vi "ReadOrWriteToJSONfile.vi"(7 "Data":T1, 8 "error in (no error)":errorcluster, 10 "Command":enum16{"Read", "Write"}(ring), 11 "JSONtext Input":string) -> (0 "error out":errorcluster, 3 "JSON text":string)   [LabVIEW 2017]
doc: "<B>This VI is used for Read or Write a JSON file.</B>"
uses:
  <vilib>/JDP Science/JSONtext/JSONtext.lvlib
  Ctrl/Property.ctl
  Ctrl/PhysicalChannel.ctl
  Ctrl/Bitfield.ctl
  Ctrl/Register.ctl
  Ctrl/ScaleType.ctl
  Ctrl/Scale.ctl
  Ctrl/EnumValue.ctl
  Ctrl/Enum.ctl
  Ctrl/Caps.ctl
  Ctrl/Data.ctl
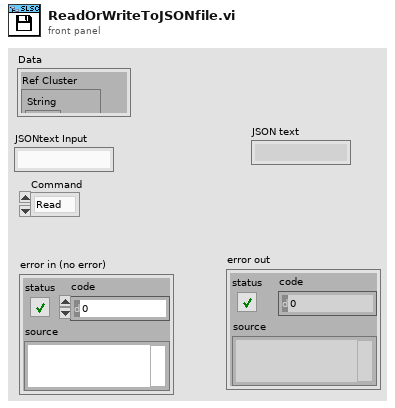
[diagram p1: front panel]
types:
  T1 = typedef "Data.ctl" = cluster{"Ref Cluster":cluster{"String":refnum<vi>, "U8":refnum<vi>, "I8":refnum<vi>, "U32":refnum<vi>, "I32":refnum<vi>, "U64":refnum<vi>, "I64":refnum<vi>, "Ring":refnum<vi>, "DBL":refnum<vi>, "Add":refnum<vi>, "Remove":refnum<vi>, "Property tree":refnum<vi>, "confirm":refnum<vi>}, "JSON Text":string, "Original JSON Text":string, "Caps":T2, "SLSC Output Tree":cluster{"Left Cell String":string, "Child Text":string[], "Child Tag":string, "Item Indent":i32, "Child Only?":bool, "Glyph Index":i32, "offline value":variant}[], "Ref Index and Control Type":cluster{"index":i32, "Datatype":string}, "Selected Type and name":cluster{"Selected Type":enum16{"Property", "Physical Channel", "Other"}, "Selected Property Name":string}, "Update whole Tree?":bool}
  T2 = typedef "Caps.ctl" = cluster{"properties":T3[], "physical channels":T4[], "registers":T5[], "scales":T7[], "enums":T9[], "productName":string}
  T3 = typedef "Property.ctl" = cluster{"name":string, "bitfield":string, "value":variant, "dataType":string, "min":variant, "max":variant, "scale":string, "access":string}
  T4 = typedef "PhysicalChannel.ctl" = cluster{"name":string, "properties":T3[]}
  T5 = typedef "Register.ctl" = cluster{"name":string, "address":i32, "size":i32, "bitfields":T6[], "initialValue":variant, "connectedProperties":string[]}
  T6 = typedef "Bitfield.ctl" = cluster{"name":string, "offset":i32, "size":i32, "signed":bool}
  T7 = typedef "Scale.ctl" = cluster{"name":string, "type":T8, "params":variant}
  T8 = typedef "ScaleType.ctl" = enum16{"NoScale", "Table", "Polynomial", "Linear"}
  T9 = typedef "Enum.ctl" = cluster{"name":string, "values":T10[]}
  T10 = typedef "EnumValue.ctl" = cluster{"name":string, "value":i32}
  T11 = enum16{"open", "replace", "create", "open or create", "replace or create", "replace or create with confirmation"}
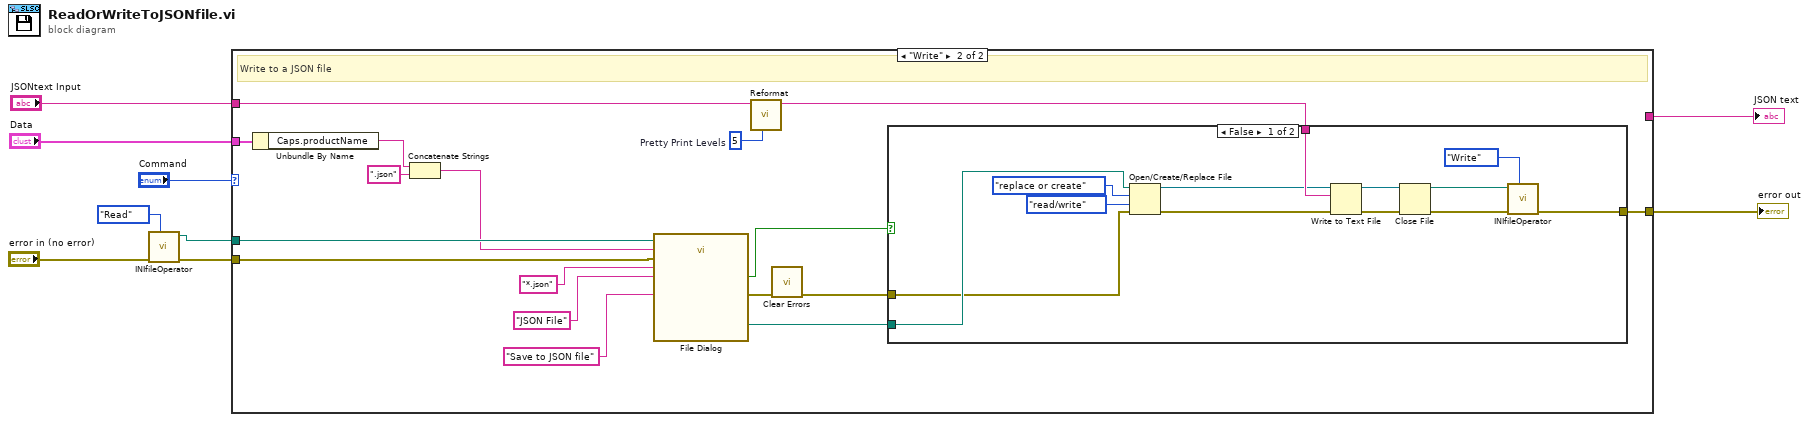
[diagram p0: block diagram]
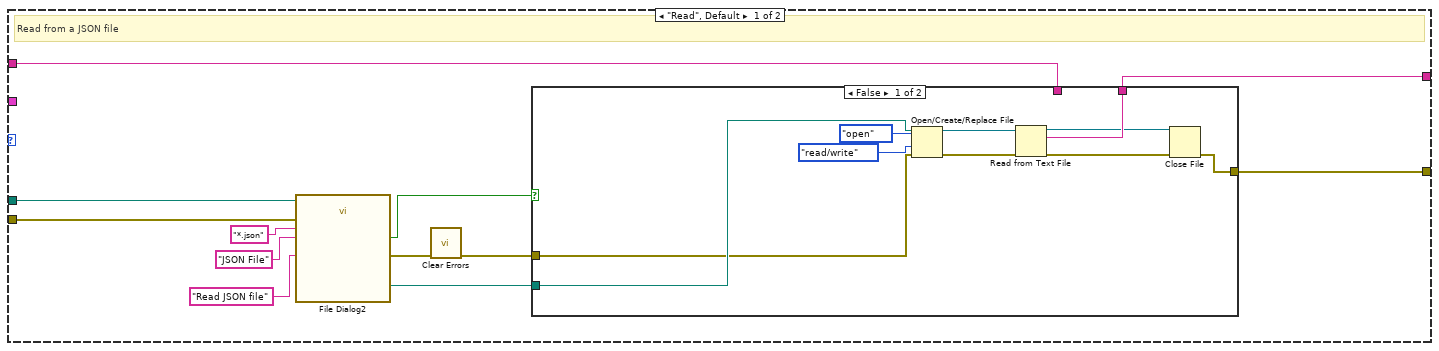
[diagram p2: hidden frame]
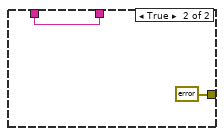
[diagram p3: hidden frame]
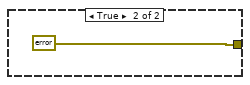
[diagram p4: hidden frame]
diagram:
  n1 = call "INIfileOperator.vi"("Command"=enum16{"Write", "Read"}."Read", "error in (no error)"="error in (no error)") -> ("error out"=w3:errorcluster, "Last Path output"=w2:path)  [unwired: 8 in]
  n2 = case shown="\"Write\"" "Command" {
    tunnel: "JSONtext Input" -> [w12 w36]
    tunnel: w2 -> [w20 w47]
    tunnel: w3 -> [w11 w45]
    tunnel: [w21 _] -> w9
    tunnel: [w13 w41] -> w8
    tunnel: "Data" -> [_ w40]
    frame "Read", Default {
      # "Read from a JSON file"
      n3 = call "File Dialog2"("start path"=w20, "prompt"="Read JSON file", "error in"=w11, "pattern (all files)"="*.json", "pattern label"="JSON File") -> ("selected path"=w10:path, "cancelled"=w14:bool, "error out"=w16:errorcluster)  [unwired: 7 in, 1 out]
      n4 = call <vilib>:"Clear Errors.vi"("error in (no error)"=w16) -> ("error out"=w15:errorcluster)  [unwired: 5 in, 1 out]
      n5 = case shown="False" w14 {
        tunnel: [w27 w32] -> w21
        tunnel: w10 -> [w26 _]
        tunnel: w15 -> [w25 _]
        tunnel: [w24 errorcluster {"status"=FALSE, "code"=0, "source"=""} ("error out")] -> w13
        tunnel: w12 -> [_ w32]
        frame False {
          n6 = Open/Create/Replace File(file path (use dialog)=w26, error in=w25, operation (0:open)=T11."open", access (0:read/write)=enum16{"read/write", "read-only", "write-only"}."read/write") -> (refnum out=w28:refnum<file>, error out=w29:errorcluster)  [unwired: 2 in, 1 out]
          n7 = Read from Text File(file (use dialog)=w28, error in=w29) -> (refnum out=w22:refnum<file>, text=w27:string, error out=w23:errorcluster)  [unwired: 2 in, 1 out]
          n8 = Close File(refnum=w22, error in=w23) -> (error out=w24:errorcluster)  [unwired: 1 out]
        }
        frame True {
        }
      }
    }
    frame "Write" {
      w34 = 5  # Pretty Print Levels
      # "Write to a JSON file"
      n9 = Unbundle By Name(w40) -> ("Caps.productName"=w39:string)
      n10 = Concatenate Strings(w39, ".json" ("string")) -> (w37:string)
      n11 = call "File Dialog"("start path"=w47, "prompt"="Save to JSON file", "default name"=w37, "error in"=w45, "pattern (all files)"="*.json", "pattern label"="JSON File") -> ("selected path"=w46:path, "cancelled"=w42:bool, "error out"=w44:errorcluster)  [unwired: 6 in, 1 out]
      n12 = call <vilib>:"Reformat.vi"("Pretty Print Levels"=w34, "JSON"=w36) -> ("<JSON>First JSON Value\n\n<JSON>"=w35:string)  [unwired: 6 in, 3 out]
      n13 = call <vilib>:"Clear Errors.vi"("error in (no error)"=w44) -> ("error out"=w43:errorcluster)  [unwired: 5 in, 1 out]
      n14 = case shown="False" w42 {
        tunnel: w35 -> [w63 _]
        tunnel: w46 -> [w58 _]
        tunnel: w43 -> [w57 _]
        tunnel: [w53 errorcluster {"status"=FALSE, "code"=0, "source"=""} ("error out")] -> w41
        frame False {
          n15 = Open/Create/Replace File(file path (use dialog)=w58, error in=w57, operation (0:open)=T11."replace or create", access (0:read/write)=enum16{"read/write", "read-only", "write-only"}."read/write") -> (refnum out=w60:refnum<file>, error out=w59:errorcluster)  [unwired: 2 in, 1 out]
          n16 = Write to Text File(file (use dialog)=w60, text=w63, error in=w59) -> (refnum out=w56:refnum<file>, error out=w55:errorcluster)  [unwired: 1 in, 1 out]
          n17 = Close File(refnum=w56, error in=w55) -> (path=w52:path, error out=w54:errorcluster)
          n18 = call "INIfileOperator.vi"("Command"=enum16{"Write", "Read"}."Write", "error in (no error)"=w54, "Last Path"=w52) -> ("error out"=w53:errorcluster)  [unwired: 7 in, 1 out]
        }
        frame True {
        }
      }
    }
  }
  "error out" <- w8
  "JSON text" <- w9
